vi "Write Loads.vi"(8 "error in (no error)":errorcluster, 10 "Loads":T1[](array[typedef]), 11 "ChromaAcLoad in":refnum<class "ChromaAcLoad.lvclass">) -> (0 "error out":errorcluster, 3 "ChromaAcLoad out":refnum<class "ChromaAcLoad.lvclass">)   [LabVIEW 2014, in "AcPwrPlugins.lvlib" / "ChromaAcLoad.lvclass"]
uses:
  ChromaAcLoad.lvclass
  TypeDefs/Load.ctl
  TypeDefs/LoadSettings.ctl
  ChromaAcLoad.lvclass/ChromaAcLoad.ctl
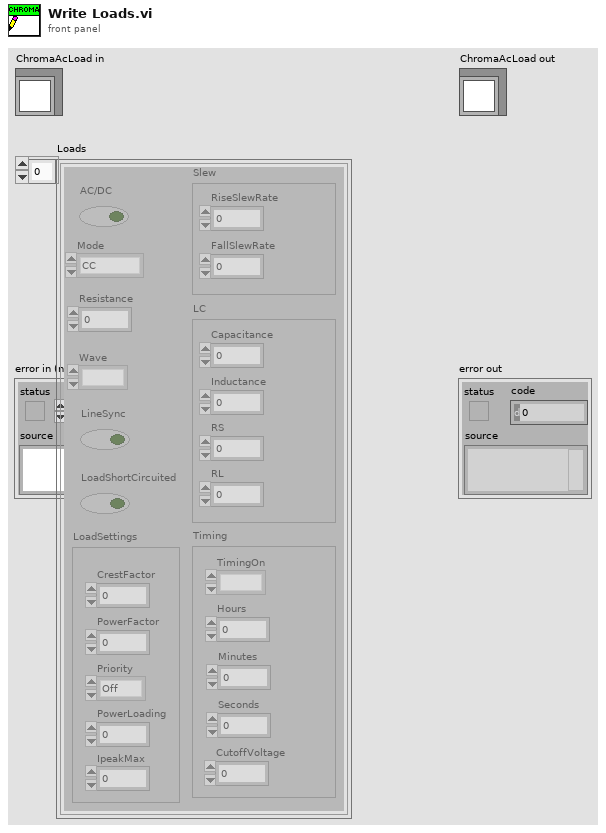
[diagram p1: front panel]
types:
  T1 = typedef "AcPwrPlugins.lvlib/ChromaAcLoad.lvclass/Load.ctl" = cluster{"AC/DC":bool, "Mode":enum16{"CC", "CP", "CR", "CV", "RLC", "RLC CP", "Inrush", "Rectified"}, "LC":cluster{"Capacitance":dbl, "Inductance":dbl, "RL":dbl, "RS":dbl}, "Resistance":dbl, "LoadSettings":T2, "Wave":enum16{""}, "LineSync":bool, "LoadShortCircuited":bool, "Slew":cluster{"RiseSlewRate":dbl, "FallSlewRate":dbl}, "Timing":cluster{"TimingOn":enum16{""}, "Hours":u32, "Minutes":u32, "Seconds":dbl, "CutoffVoltage":dbl}}
  T2 = typedef "AcPwrPlugins.lvlib/ChromaAcLoad.lvclass/LoadSettings.ctl" = cluster{"CrestFactor":dbl, "PowerFactor":dbl, "PowerLoading":dbl, "IpeakMax":dbl, "Priority":enum16{"Off", "Hold Up", "Transfer"}}
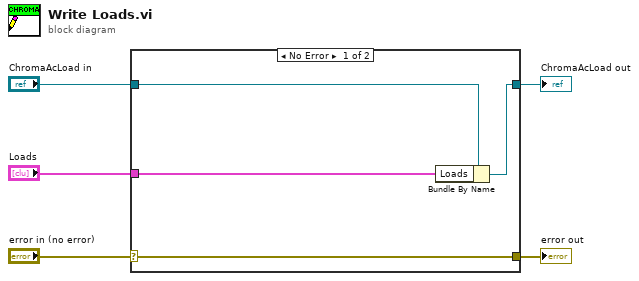
[diagram p0: block diagram]
diagram:
  n1 = case shown="No Error" "error in (no error)" {
    selector: "error in (no error)" -> [w9 w10]
    tunnel: [w9 w10] -> w4
    tunnel: [w7 w11] -> w2
    tunnel: "ChromaAcLoad in" -> [w8 w11]
    tunnel: "Loads" -> [w6 _]
    frame No Error {
      n2 = Bundle By Name(cluster=w8, "Loads"=w6) -> (w7:refnum<class "ChromaAcLoad.lvclass">)
    }
    frame Error {
    }
  }
  "error out" <- w4
  "ChromaAcLoad out" <- w2
